vi "Auto Discovery.vi"(7 "Instr Selection":T1(ring), 8 "error in (no error)":errorcluster, 11 "BH Druck PACE Series in":refnum<class "BH Druck PACE Series.lvclass">) -> (0 "error out":errorcluster, 1 "Connected PACE Device":refnum<visa-resource-name>[](array[refnum]), 2 "Selected Instrument":refnum<visa-resource-name>, 3 "BH Druck PACE Series out":refnum<class "BH Druck PACE Series.lvclass">, 10 "Connected Instrument":string[](array[string]))   [LabVIEW 2022 SP3, in "BH Druck PACE Series.lvclass"]
uses:
  BH Druck PACE Series.lvclass
  <vilib>/Instr/_visa.llb/VISA Find Search Mode.ctl
  BH Druck PACE Series.lvclass/BH Druck PACE Series.ctl
  <vilib>/regexp/Match Regular Expression.xnode
panel:
  in  "VISA resource name Input":refnum<visa-resource-name>
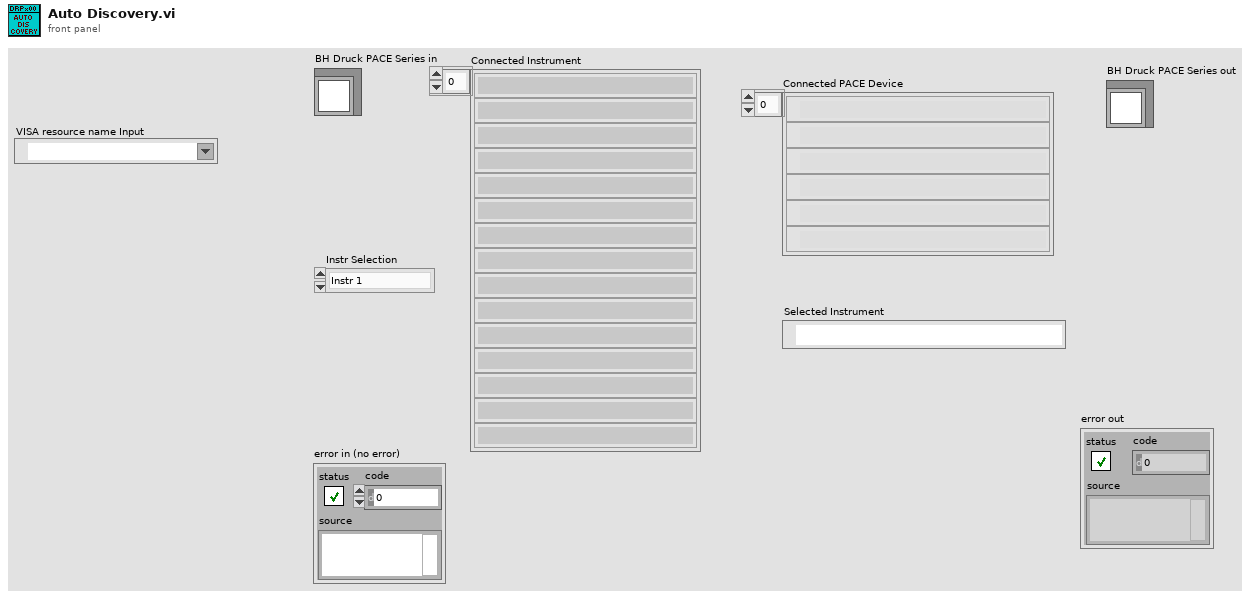
[diagram p1: front panel]
types:
  T1 = enum16{"Instr 1", "Instr 2", "Instr 3", "Instr 4", "Instr 5", "Instr 6", "Instr 7", "Instr 8", "Instr 9", "Instr 10", "Instr 11", "Instr 12", "Instr 13", "Instr 14", "Instr 15", "Instr 16", "Instr 17", "Instr 18", "Instr 19", "Instr 20"}
  T2 = typedef "VISA Find Search Mode.ctl" = u32
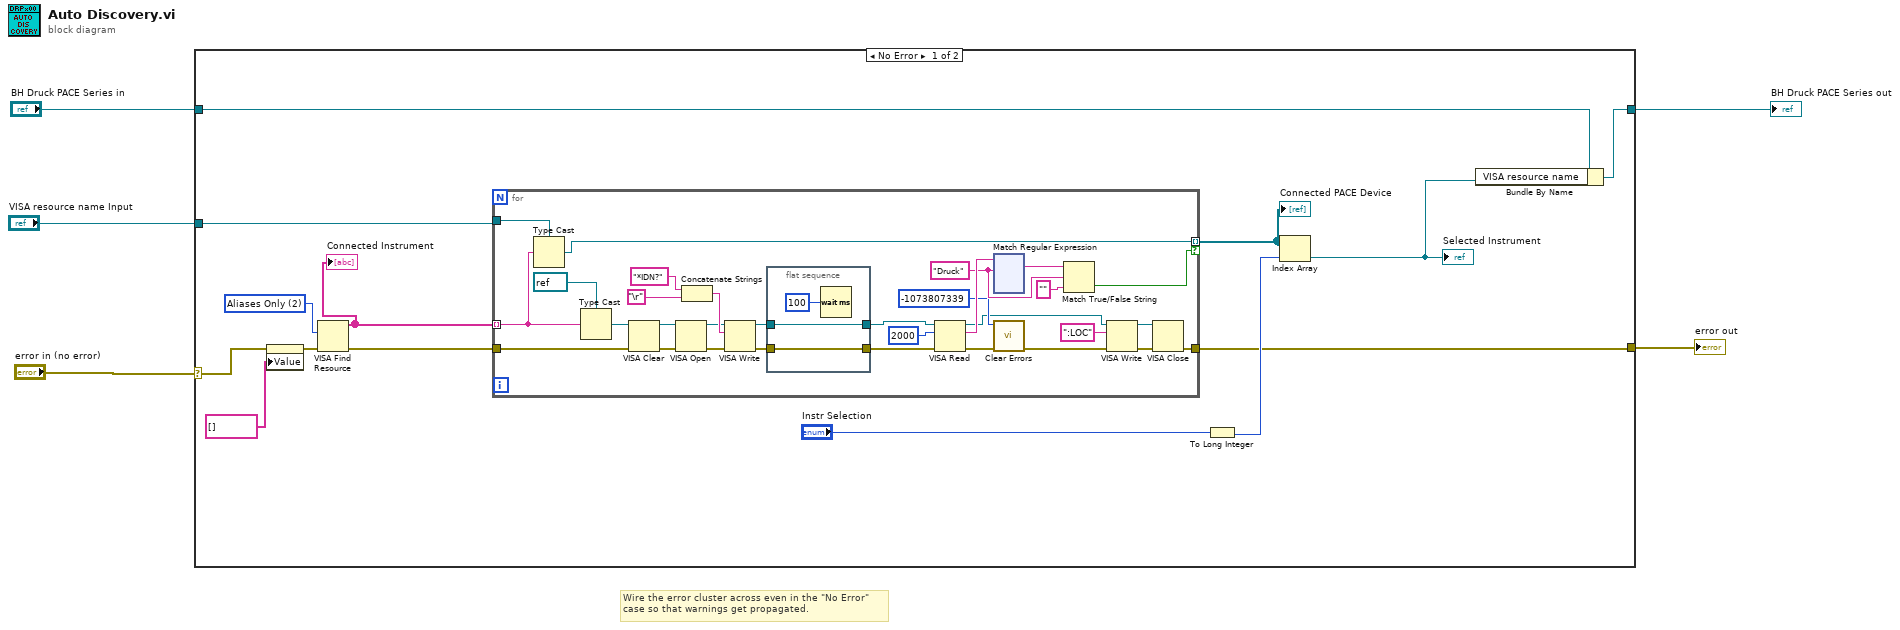
[diagram p0: block diagram]
diagram:
  # "Wire the error cluster across even in the \"No Error\"\ncase so that warnings get propagated."
  n1 = case shown="No Error" "error in (no error)" {
    selector: "error in (no error)" -> [w11 w172]
    tunnel: [w10 w172] -> w4
    tunnel: [w6 w171] -> w2
    tunnel: "BH Druck PACE Series in" -> [w7 w171]
    tunnel: "VISA resource name Input" -> [w9 _]
    frame No Error {
      w12 = T2 2 items=["Canonical Names Only"=0, "Aliases Only"=2, "Include Matching Aliases"=3, "Include All Aliases"=4] ("Search Mode")
      n2 = property on="Connected Instrument" class="Arr (strict)"(error in=w11, "Value"=string[] []) -> (error out=w19:errorcluster)  [unwired: 1 in, 1 out]
      n3 = VISA Find Resource(8:w19, 10:w12) -> (0:w15:errorcluster, 3:w14:string[])  [unwired: 1 in, 1 out]
      "Connected Instrument" <- w14
      n4 = for {
        tunnel: w14 -> [w40] mode=indexing
        tunnel: w15 -> [w25]
        tunnel: w9 -> [w41]
        tunnel: [w35] -> w16 mode=indexing if=w34
        tunnel: [w33] -> w10
        w37 = "Druck" ("true string")
        n5 = Type Cast(type=w41, x=w40) -> (*(type *) &x=w35:refnum<visa-resource-name>)
        n6 = Type Cast(type=refnum<visa-resource-name> refnum ("VISA resource name"), x=w40) -> (*(type *) &x=w24:refnum<visa-resource-name>)
        n7 = VISA Clear(VISA resource name=w24, error in (no error)=w25) -> (VISA resource name out=w23:refnum<visa-resource-name>, error out=w22:errorcluster)
        n8 = VISA Open(error in (no error)=w22, VISA resource name=w23) -> (VISA resource name=w21:refnum<visa-resource-name>, error out=w20:errorcluster)  [unwired: 3 in]
        n9 = Concatenate Strings("*IDN?", "\r") -> (w47:string)
        n10 = VISA Write(VISA resource name=w21, write buffer=w47, error in (no error)=w20) -> (VISA resource name out=w46:refnum<visa-resource-name>, error out=w45:errorcluster)  [unwired: 1 out]
        n11 = flat-sequence {
          tunnel: w46 -> [w169]
          tunnel: w45 -> [w168]
          tunnel: [w169] -> w43
          tunnel: [w168] -> w44
          frame #0 {
            n12 = Wait (ms)(milliseconds to wait=u32 100) -> ()  [unwired: 1 out]
          }
        }
        n13 = VISA Read(VISA resource name=w43, byte count=u32 2000, error in (no error)=w44) -> (VISA resource name out=w29:refnum<visa-resource-name>, read buffer=w39:string, error out=w31:errorcluster)  [unwired: 1 out]
        n14 = xnode "Match Regular Expression"("input string"=w39, "regular expression"=w37) -> ("whole match"=w38:string)  [unwired: 4 in, 4 out]
        n15 = call <vilib>:"Clear Errors.vi"("error in (no error)"=w31, "specific error code to clear (0: all)"=-1073807339) -> ("error out"=w30:errorcluster)  [unwired: 4 in, 1 out]
        n16 = Match True/False String(2:"" ("false string"), 3:w37, 4:w38) -> (0:w34:bool)  [unwired: 1 out]
        n17 = VISA Write(VISA resource name=w29, write buffer=":LOC", error in (no error)=w30) -> (VISA resource name out=w27:refnum<visa-resource-name>, error out=w28:errorcluster)  [unwired: 1 out]
        n18 = VISA Close(VISA resource name=w27, error in (no error)=w28) -> (error out=w33:errorcluster)
      }
      "Connected PACE Device" <- w16
      n19 = To Long Integer(number="Instr Selection") -> (32bit integer=w18:i32)
      n20 = Index Array(array=w16, index=w18) -> (element=w8:refnum<visa-resource-name>)
      "Selected Instrument" <- w8
      n21 = Bundle By Name(cluster=w7, "VISA resource name"=w8) -> (w6:refnum<class "BH Druck PACE Series.lvclass">)
    }
    frame Error {
    }
  }
  "error out" <- w4
  "BH Druck PACE Series out" <- w2
